vi "PathPlanner_RotationTarget_ForSegmentIndex.vi"(9 "SegmentIndex":i32, 11 "RotationTarget":T1={"target"={"VALUE"=0.0, "COS"=1.0, "SIN"=0.0}, "WaypointRelativePosition"=0.0, "Exists"=FALSE} {"target"."SIN" format="%13.4f"; "target"."COS" format="%13.4f"; "target"."VALUE" format="%13.4f"}) -> (3 "new RotationTarget":T1={"target"={"VALUE"=0.0, "COS"=1.0, "SIN"=0.0}, "WaypointRelativePosition"=0.0, "Exists"=FALSE} {"target"."SIN" format="%13.4f"; "target"."COS" format="%13.4f"; "target"."VALUE" format="%13.4f"})   [LabVIEW 2019, in "PathPlanner24.lvlib"]
uses:
  PathPlanner24.lvlib
  TypeDef/PathPlannerRotationTarget.ctl
  <vilib>/Rock Robotics/WPI/ThirdParty/JAS_Junk/TrajLib/TypeDef/ROTATION2D.ctl
  <vilib>/Rock Robotics/WPI/ThirdParty/JAS_Junk/TrajLib/Trajectory_Library.lvlib
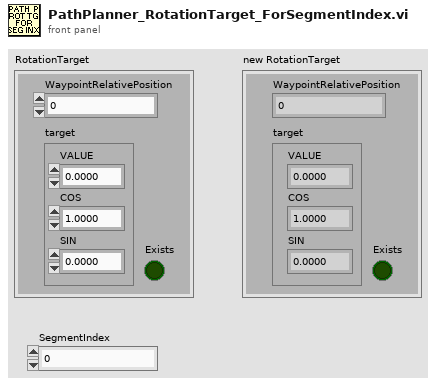
[diagram p1: front panel]
types:
  T1 = typedef "PathPlanner24.lvlib/PathPlannerRotationTarget.ctl" = cluster{"target":T2, "WaypointRelativePosition":dbl, "Exists":bool}
  T2 = typedef "Trajectory_Library.lvlib/ROTATION2D.ctl" = cluster{"VALUE":dbl, "COS":dbl, "SIN":dbl}
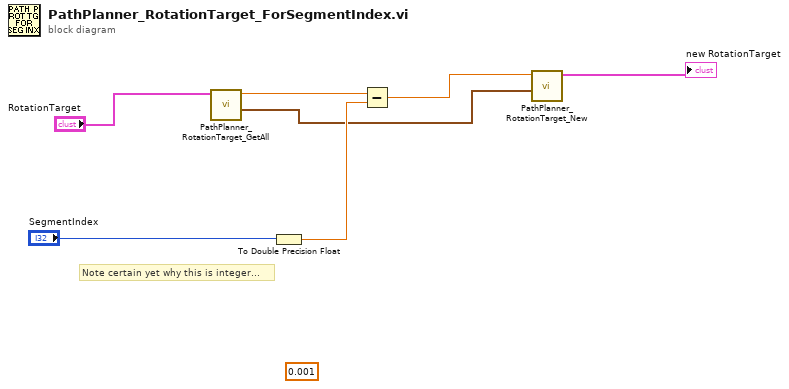
[diagram p0: block diagram]
diagram:
  (unwired) 0.001 ("y")
  # "Note certain yet why this is integer..."
  n1 = call "PathPlanner_RotationTarget_GetAll.vi"("RotationTarget"="RotationTarget") -> ("target"=w3:T2, "WaypointRelativePosition"=w5:dbl)  [unwired: 9 in]
  n2 = To Double Precision Float(number="SegmentIndex") -> (double precision float=w4:dbl)
  n3 = Subtract(x=w5, y=w4) -> (x-y=w2:dbl)
  n4 = call "PathPlanner_RotationTarget_New.vi"("target"=w3, "WaypointRelativePosition"=w2) -> ("RotationTarget"=→"new RotationTarget":T1)  [unwired: 9 in]
